vi "Stop Aquisition.vi"(8 "error in (no error)":errorcluster, 11 "DAQ Process in":refnum<class "DAQ Process.lvclass">) -> (0 "error out":errorcluster, 3 "DAQ Process out":refnum<class "DAQ Process.lvclass">)   [LabVIEW 2022 SP3, in "DAQ Process.lvlib" / "DAQ Process.lvclass"]
uses:
  DAQ Process.lvclass
  DAQ Process.lvclass/DAQ Process.ctl
  XY Stage/Process Actor/Process Framework/Process State Data/Process State Data.lvclass
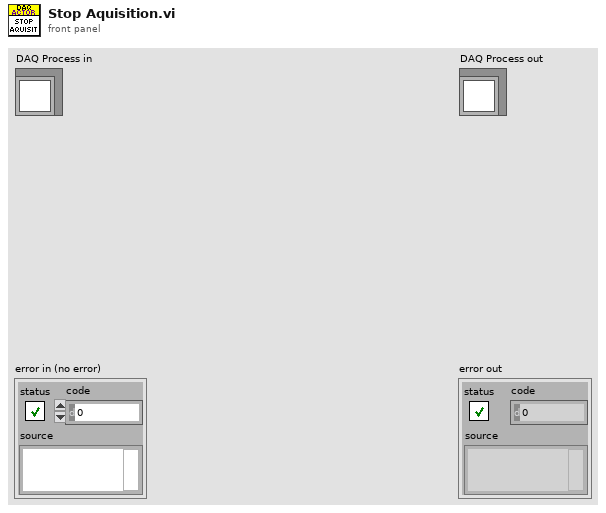
[diagram p1: front panel]
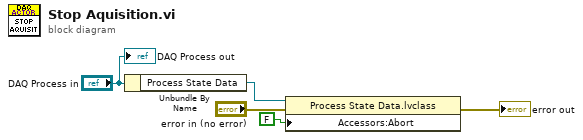
[diagram p0: block diagram]
diagram:
  n1 = Unbundle By Name("DAQ Process in") -> ("Process State Data"=w4:refnum<data-value>)
  n2 = property class="Process State Data.lvclass"(reference=w4, error in="error in (no error)", "Accessors:Abort"=FALSE ("Abort")) -> (error out=→"error out":errorcluster)  [unwired: 1 out]
  "DAQ Process out" <- "DAQ Process in"
